vi "Charge and Discharge State Machine VI.vi"() -> ()   [LabVIEW 2017]
uses:
  Downloads/VVWRA HMM/Globals.vi
panel:
  out "Refresh Battery SOC (%)":u8
  out "Power Needed (kW)":i32
  out "Refresh Battery Power (kW)":i32
  out "Discharge Battery Power (kW)":i32
  out "Discharge State":T1(ring)
  out "SCE_Power (kW)":i32
  out "Charge State":T1(ring)
  out "Discharging Battery SOC (%)":u8
  out "Charging Battery SOC (%)":u8
  out "Charge Battery Power (kW)":i32
  in  "Stop Button":bool
  # "Contact information: \nMatthew Scudder\nmatthew.scudderr@gmail.com\n773-306-9466"
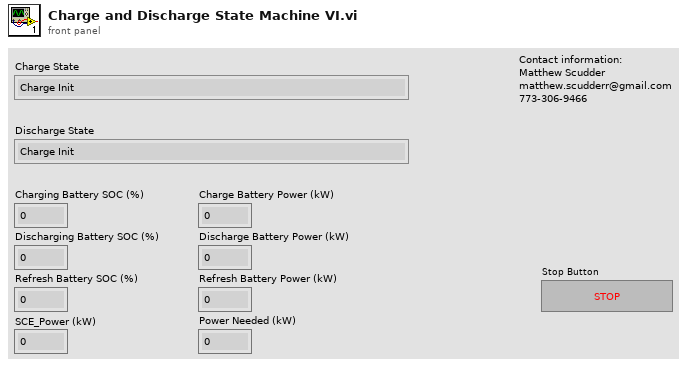
[diagram p1: front panel]
types:
  T1 = enum16{"Charge Init", "Start Charging Loop", "Check SOC < 75%", "Charge_Bat Power > -86 kW", "Charge_Bat Power = -86 kW", "Charge_Bat Power > -10 kW", "Discharge_Bat Power >= 40 kW && SCE_Power >= 110 kW", "Charge_Bat Power = Charge_Bat Power + 20kW", "Charge_Bat Power = 0 kW", "Wait for Discharge_Bat SOC", "Discharge Init", "Start Discharging Loop", "SCE_Power < 90 kW_1", "Discharge_Bat SOC < 25%_1", "Charge_Bat SOC >= 75%", "Battery Role Change", "SCE_Power < 95 kW_1", "Refresh_Bat Power = Refresh_Bat Power + 5 kW", "Refresh_Bat Power >= 100 kW", "Refresh_Bat SOC < 10%", "Refresh_Bat = Charge_Bat", "Power_Needed = 95 kW - SCE_Power", "Discharge_Bat Power - Power_Needed < -86 kW", "Alarm Discharge_Bat Can't Meet Demand", "Discharge_Bat Power = Discharge_Bat Power - Power_Needed", "SCE_Power < 90 kW_2", "SCE_Power < 95 kW_2", "Discharge_Bat Power = Discharge_Bat Power + 5 kW", "SCE_Power < 90 kW_3", "Discharge_Bat Power >= 40 kW", "Discharge_Bat SOC < 25%_2", "Shutdown"}
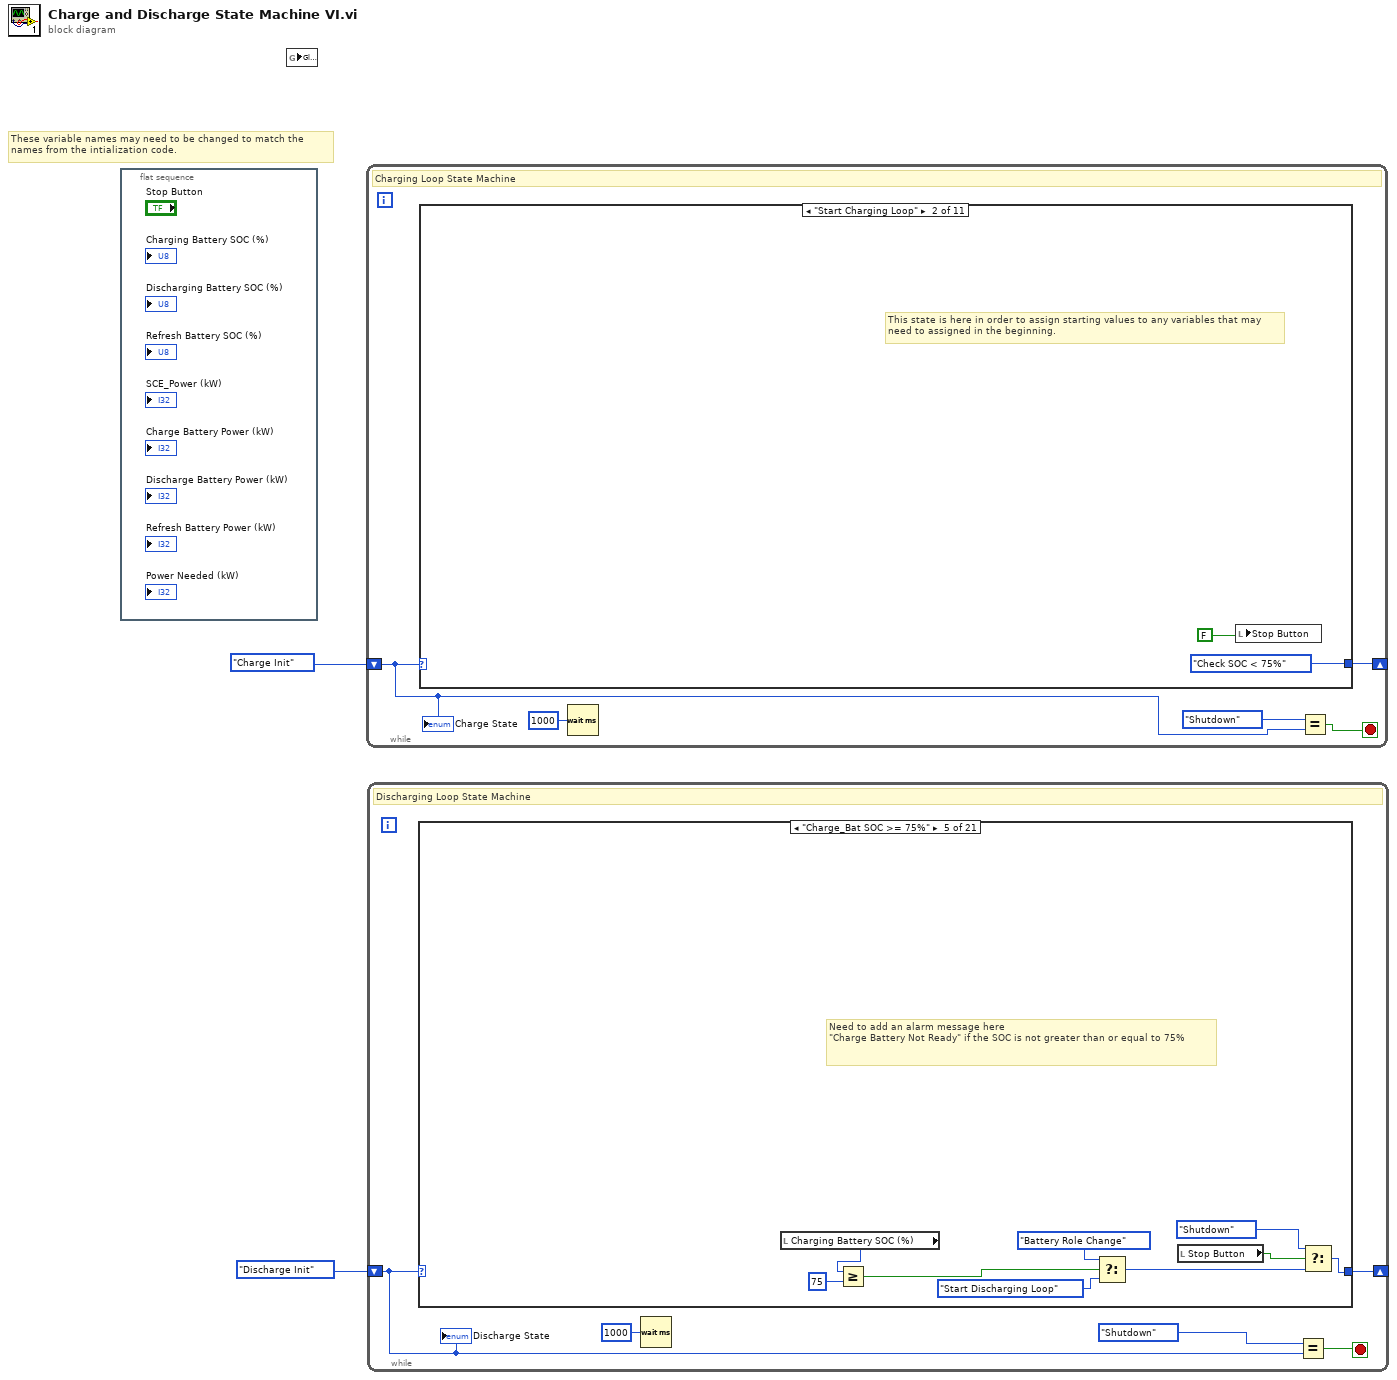
[diagram p0: block diagram]
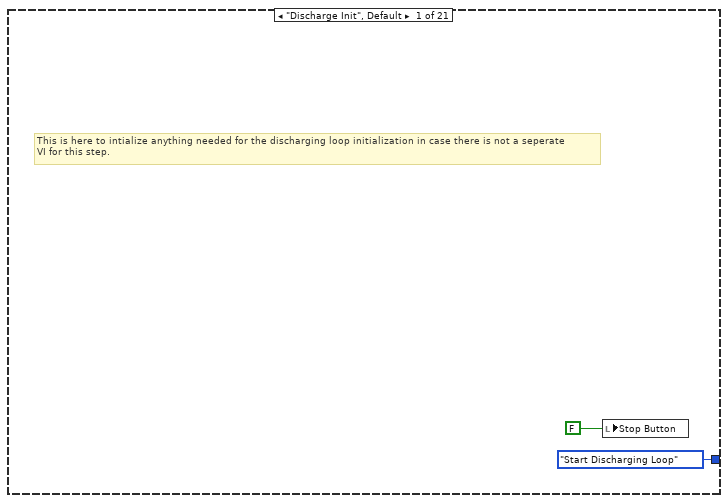
[diagram p2: hidden frame]
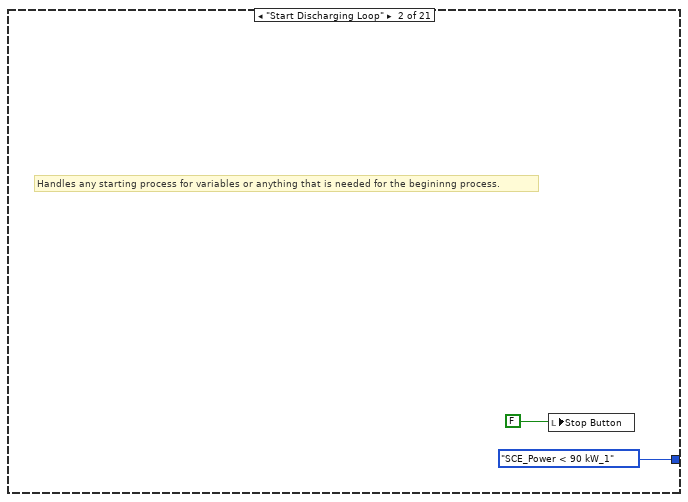
[diagram p3: hidden frame]
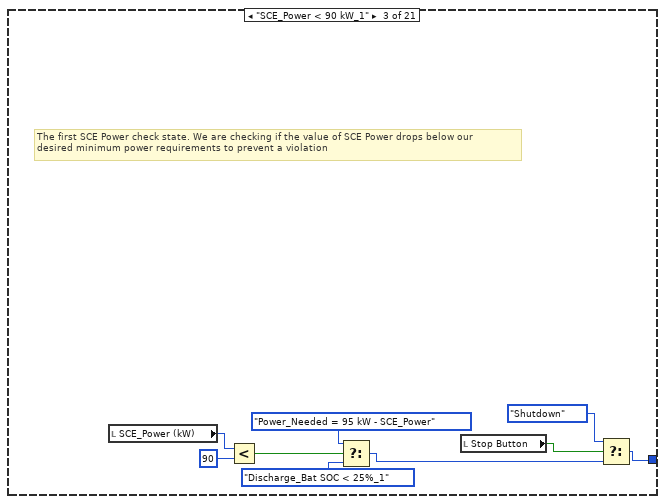
[diagram p4: hidden frame]
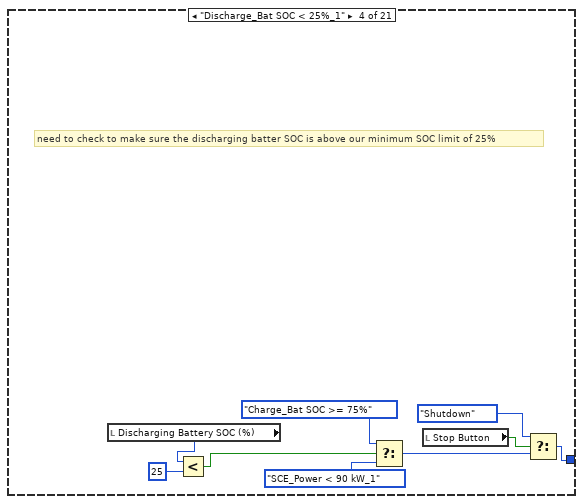
[diagram p5: hidden frame]
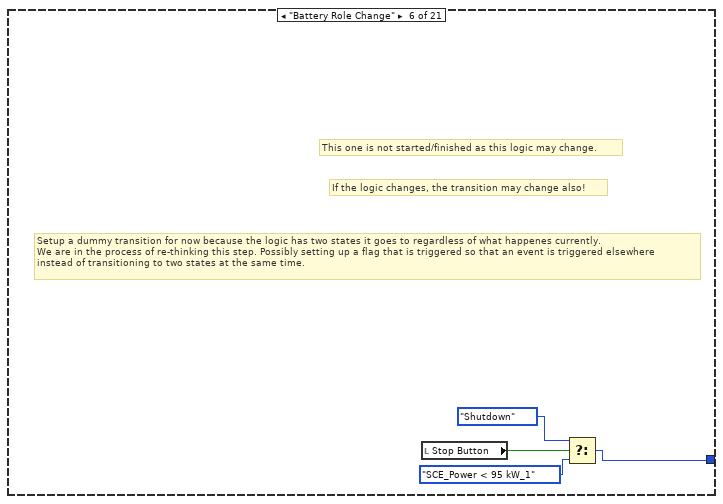
[diagram p6: hidden frame]
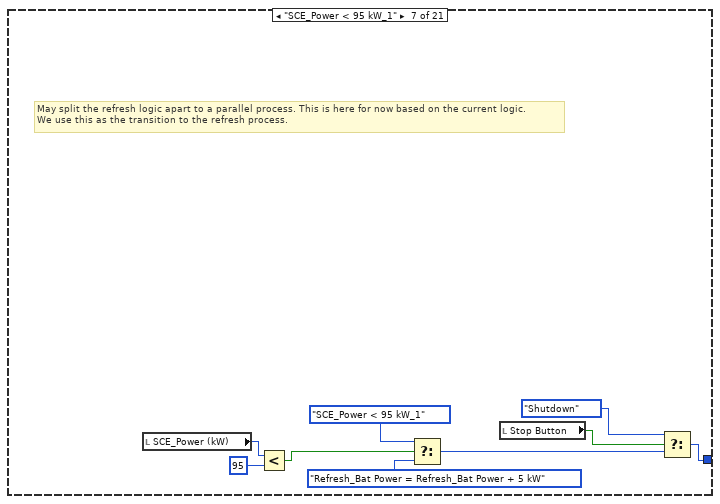
[diagram p7: hidden frame]
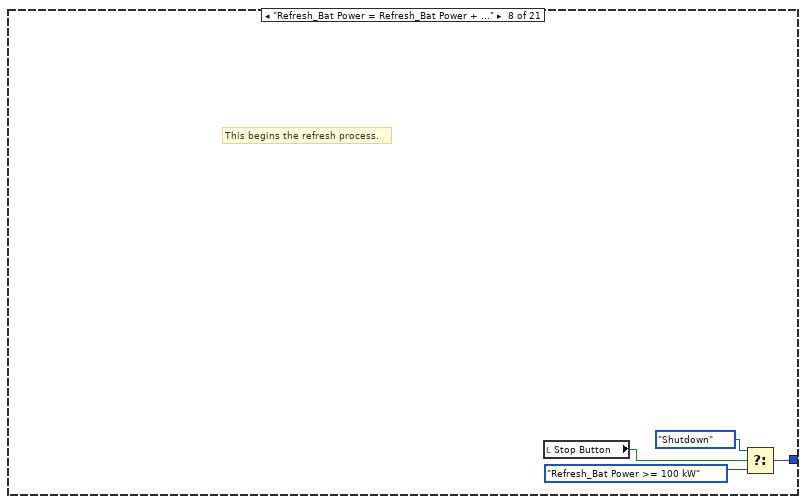
[diagram p8: hidden frame]
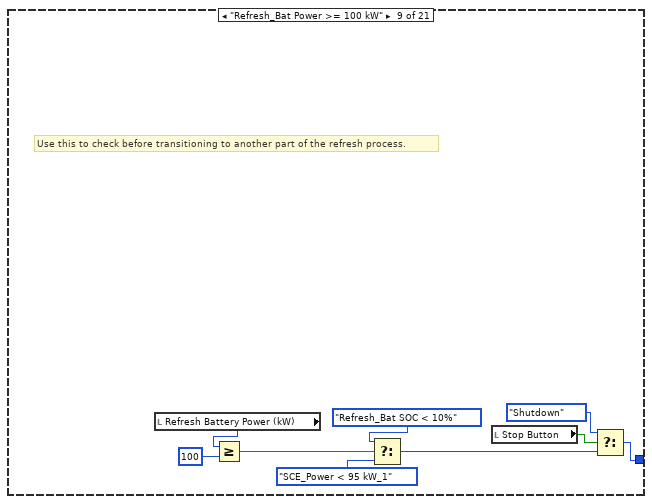
[diagram p9: hidden frame]
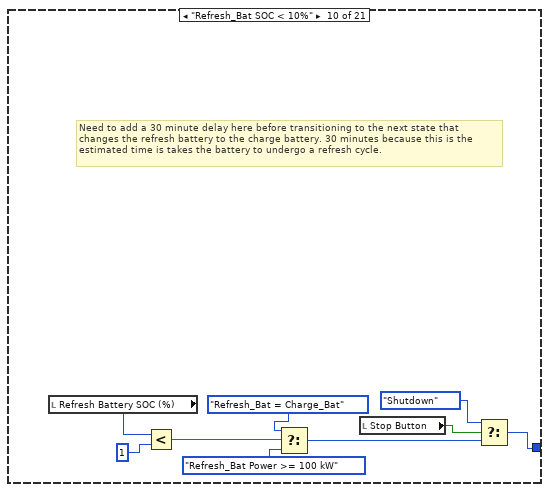
[diagram p10: hidden frame]
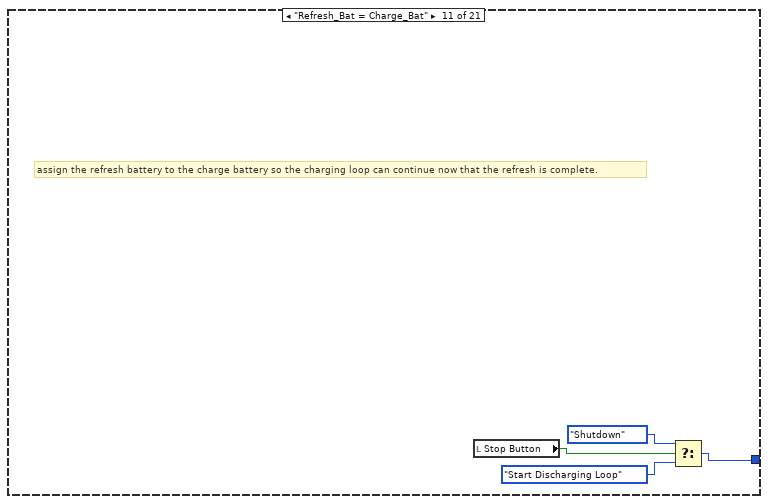
[diagram p11: hidden frame]
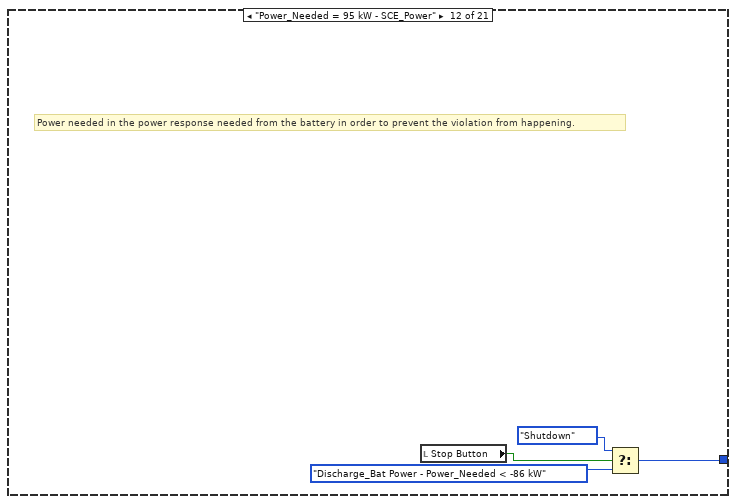
[diagram p12: hidden frame]
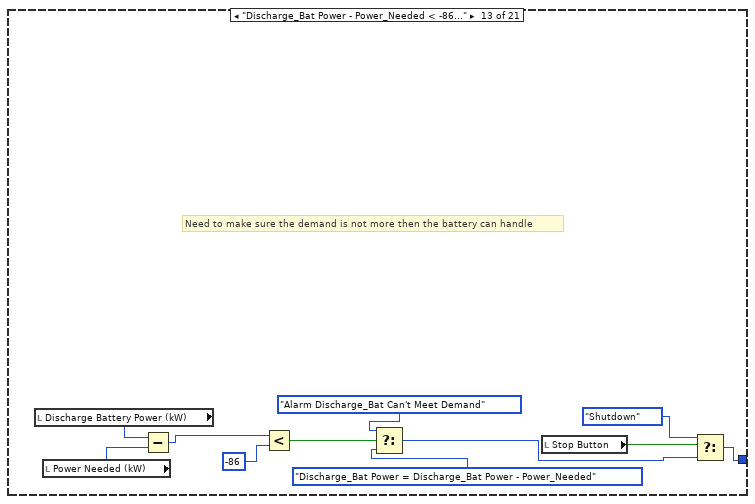
[diagram p13: hidden frame]
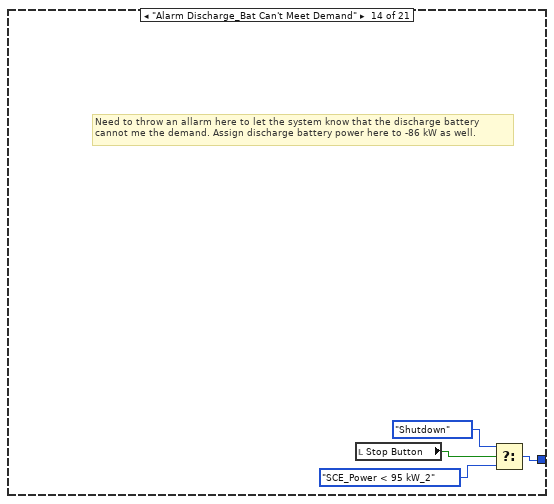
[diagram p14: hidden frame]
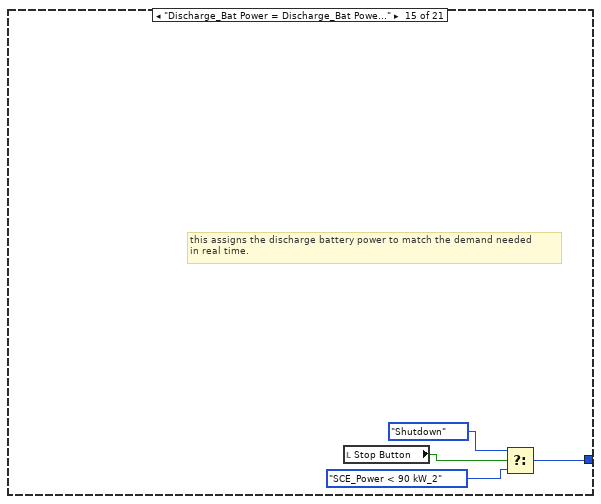
[diagram p15: hidden frame]
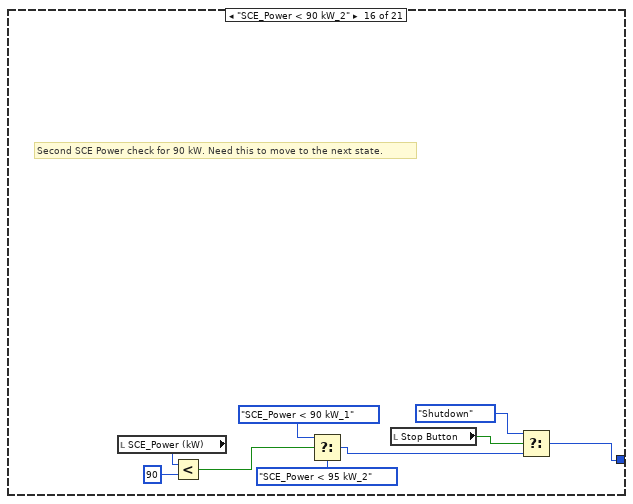
[diagram p16: hidden frame]
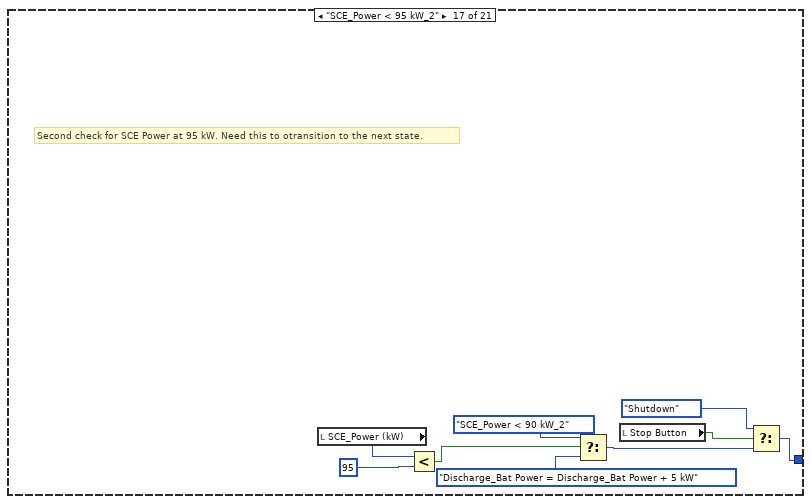
[diagram p17: hidden frame]
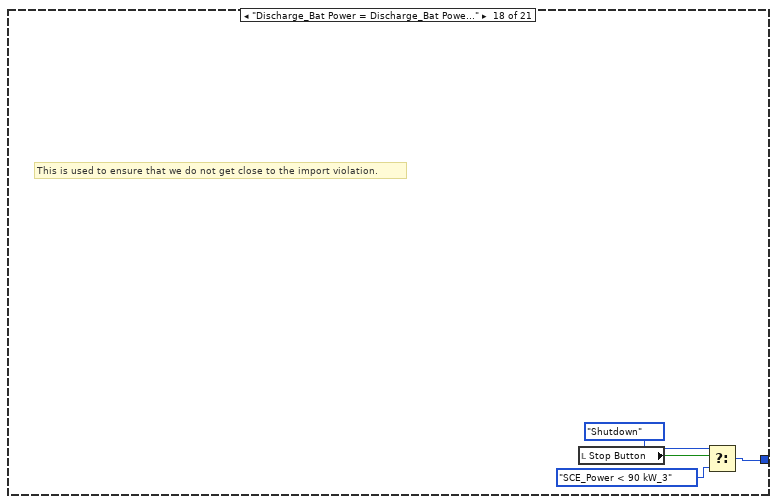
[diagram p18: hidden frame]
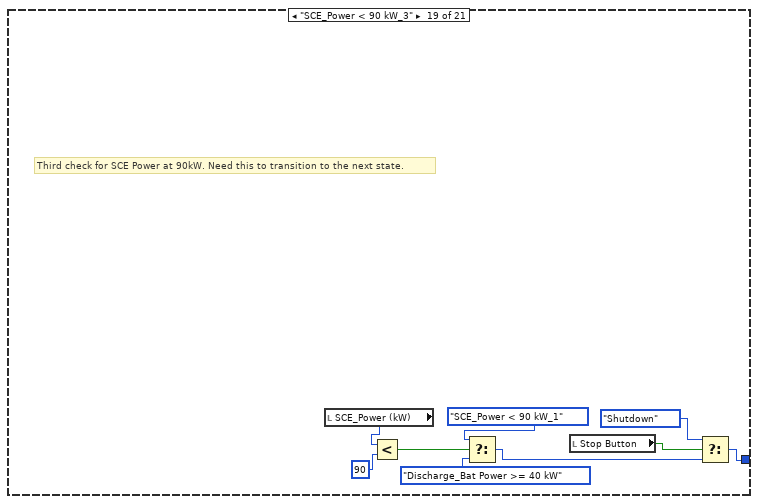
[diagram p19: hidden frame]
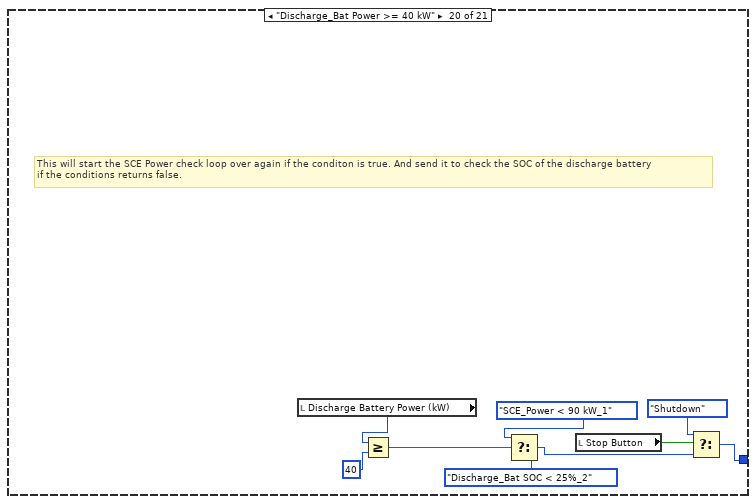
[diagram p20: hidden frame]
diagram:
  # "These variable names may need to be changed to match the \nnames from the intialization code."
  n1 = flat-sequence {
    frame #0 {
    }
  }
  n2 = global read "Globals.vi" item#-1() -> ()  [unwired: 1 in]
  n3 = while {
    shift-right: [w4] -> _
    shift-left: T1."Charge Init" ("States") -> [w5]
    stop <- w7 stop-if-true
    # "Charging Loop State Machine"
    n4 = case shown="\"Start Charging Loop\"" w5 {
      tunnel: [T1."Start Charging Loop" ("States") T1."Check SOC < 75%" ("States") w15 w22 w30 w34 w43 w59 w63 w72 T1."Shutdown" ("States")] -> w4
      frame "Charge Init", Default {
        # "Any Communication between the controller and the Inverters is done through a MODBUS Serial connection.\nThe inverter register values are in hex."
        # "Any communication between the controller and the BMS is done through MODBUS TCP/IP.\nThe BMS register values are in decimal."
        # "initialization code goes here. Either we use a subVI for the intitialization of the hardware or we \ninput the intialization code here."
        n5 = local write "Stop Button"(FALSE) -> ()
      }
      frame "Start Charging Loop" {
        # "This state is here in order to assign starting values to any variables that may\nneed to assigned in the beginning."
        n6 = local write "Stop Button"(FALSE) -> ()
      }
      frame "Check SOC < 75%" {
        # "We need to read in values of the battery that is currently assigned to charge. This is done using MODBUS TCP/IP\nbetween our controller and the BMS of the charging battery. The maximum allowed SOC is 75%"
        n7 = local read "Charging Battery SOC (%)"() -> (w20:u8)
        n8 = Less?(x=w20, y=u8 75) -> (x < y?=w18:bool)
        n9 = Select(t=T1."Charge_Bat Power > -86 kW" ("States"), s=w18, f=T1."Charge_Bat Power > -10 kW" ("States")) -> (s? t:f=w13:T1)
        n10 = local read "Stop Button"() -> (w12:bool)
        n11 = Select(t=T1."Shutdown" ("States"), s=w12, f=w13) -> (s? t:f=w15:T1)
      }
      frame "Charge_Bat Power > -86 kW" {
        # "We need the charging battery output power to be set to -86 kW here because of the requirements of the \ntypes of batteries that we are working with.\nThis is used to keep the battery within the SOC limit range of 25%-75%"
        n12 = local read "Charge Battery Power (kW)"() -> (w25:i32)
        n13 = Greater?(x=w25, y=-86) -> (0:w24:bool)
        n14 = Select(t=T1."Charge_Bat Power = -86 kW" ("States"), s=w24, f=T1."Check SOC < 75%" ("States")) -> (s? t:f=w26:T1)
        n15 = local read "Stop Button"() -> (w21:bool)
        n16 = Select(t=T1."Shutdown" ("States"), s=w21, f=w26) -> (s? t:f=w22:T1)
      }
      frame "Charge_Bat Power = -86 kW" {
        # "We need to discharge the battery to 75% SOC if it is over 75% SOC"
        n17 = local read "Stop Button"() -> (w33:bool)
        n18 = Select(t=T1."Shutdown" ("States"), s=w33, f=T1."Check SOC < 75%" ("States")) -> (s? t:f=w30:T1)
      }
      frame "Charge_Bat Power > -10 kW" {
        # "We use this check to either send the battery into a dwell state that waits for the discharge battery \nor another check that compares both the SCE power and discharge battery output"
        n19 = local read "Charge Battery Power (kW)"() -> (w42:i32)
        n20 = Greater?(x=w42, y=-10) -> (0:w40:bool)
        n21 = Select(t=T1."Charge_Bat Power = 0 kW" ("States"), s=w40, f=T1."Discharge_Bat Power >= 40 kW && SCE_Power >= 110 kW" ("States")) -> (s? t:f=w37:T1)
        n22 = local read "Stop Button"() -> (w36:bool)
        n23 = Select(t=T1."Shutdown" ("States"), s=w36, f=w37) -> (s? t:f=w34:T1)
      }
      frame "Discharge_Bat Power >= 40 kW && SCE_Power >= 110 kW" {
        # "We need to check if both the SCE Power and Discharge Battery Power conditions are met in order\nto move to the next state. We will continue to stay in this state until the conditions are met"
        n24 = local read "Discharge Battery Power (kW)"() -> (w55:i32)
        n25 = local read "SCE_Power (kW)"() -> (w52:i32)
        n26 = Greater Or Equal?(x=w55, y=40) -> (x >= y?=w53:bool)
        n27 = Greater Or Equal?(x=w52, y=110) -> (x >= y?=w50:bool)
        n28 = And(x=w53, y=w50) -> (x .and. y?=w49:bool)
        n29 = Select(t=T1."Charge_Bat Power = Charge_Bat Power + 20kW" ("States"), s=w49, f=T1."Discharge_Bat Power >= 40 kW && SCE_Power >= 110 kW" ("States")) -> (s? t:f=w46:T1)
        n30 = local read "Stop Button"() -> (w45:bool)
        n31 = Select(t=T1."Shutdown" ("States"), s=w45, f=w46) -> (s? t:f=w43:T1)
      }
      frame "Charge_Bat Power = Charge_Bat Power + 20kW" {
        # "Need add a 30 delay here before moving onto the next state"
        n32 = local read "Stop Button"() -> (w56:bool)
        n33 = Select(t=T1."Shutdown" ("States"), s=w56, f=T1."Charge_Bat Power > -10 kW" ("States")) -> (s? t:f=w59:T1)
      }
      frame "Charge_Bat Power = 0 kW" {
        # "We need to set the charging battery to zerro output and input in order to wait for the discharging battery SOC"
        n34 = local read "Stop Button"() -> (w60:bool)
        n35 = Select(t=T1."Shutdown" ("States"), s=w60, f=T1."Wait for Discharge_Bat SOC" ("States")) -> (s? t:f=w63:T1)
      }
      frame "Wait for Discharge_Bat SOC" {
        # "The charging loop can begin again once the discharging battery reaches 0% SOC making the discharge battery \nswitch to the refresh battery and the charging battery switch to a discharging battery."
        n36 = local read "Discharging Battery SOC (%)"() -> (w66:u8)
        n37 = Equal?(x=w66, y=u8 0) -> (x = y?=w64:bool)
        n38 = Select(t=T1."Start Charging Loop" ("States"), s=w64, f=T1."Wait for Discharge_Bat SOC" ("States")) -> (s? t:f=w69:T1)
        n39 = local read "Stop Button"() -> (w70:bool)
        n40 = Select(t=T1."Shutdown" ("States"), s=w70, f=w69) -> (s? t:f=w72:T1)
      }
      frame "Shutdown" {
        # "Have this state in cause the system needs to be shut down in a certain order as to save any variable data that would be \nnecessary for the initialzation of the program once booted up again."
      }
    }
    n41 = Wait (ms)(milliseconds to wait=u32 1000) -> ()  [unwired: 1 out]
    n42 = Equal?(x=T1."Shutdown" ("States"), y=w5) -> (x = y?=w7:bool)
    "Charge State" <- w5
  }
  n43 = while {
    shift-right: [w75] -> _
    shift-left: T1."Discharge Init" ("States") -> [w77]
    stop <- w78 stop-if-true
    # "Discharging Loop State Machine"
    n44 = case shown="\"Charge_Bat SOC >= 75%\"" w77 {
      tunnel: [T1."Start Discharging Loop" ("States") T1."SCE_Power < 90 kW_1" ("States") w83 w92 w102 w113 w114 w123 w127 w136 w145 w152 w153 w167 w171 w172 w181 w190 w194 w203 w212] -> w75
      frame "Discharge Init", Default {
        # "This is here to intialize anything needed for the discharging loop initialization in case there is not a seperate\nVI for this step."
        n45 = local write "Stop Button"(FALSE) -> ()
      }
      frame "Start Discharging Loop" {
        # "Handles any starting process for variables or anything that is needed for the begininng process."
        n46 = local write "Stop Button"(FALSE) -> ()
      }
      frame "SCE_Power < 90 kW_1" {
        # "The first SCE Power check state. We are checking if the value of SCE Power drops below our \ndesired minimum power requirements to prevent a violation"
        n47 = local read "SCE_Power (kW)"() -> (w91:i32)
        n48 = Less?(x=w91, y=90) -> (x < y?=w89:bool)
        n49 = Select(t=T1."Power_Needed = 95 kW - SCE_Power" ("States"), s=w89, f=T1."Discharge_Bat SOC < 25%_1" ("States")) -> (s? t:f=w86:T1)
        n50 = local read "Stop Button"() -> (w85:bool)
        n51 = Select(t=T1."Shutdown" ("States"), s=w85, f=w86) -> (s? t:f=w83:T1)
      }
      frame "Discharge_Bat SOC < 25%_1" {
        # "need to check to make sure the discharging batter SOC is above our minimum SOC limit of 25%"
        n52 = local read "Discharging Battery SOC (%)"() -> (w100:u8)
        n53 = Less?(x=w100, y=u8 25) -> (x < y?=w98:bool)
        n54 = Select(t=T1."Charge_Bat SOC >= 75%" ("States"), s=w98, f=T1."SCE_Power < 90 kW_1" ("States")) -> (s? t:f=w95:T1)
        n55 = local read "Stop Button"() -> (w94:bool)
        n56 = Select(t=T1."Shutdown" ("States"), s=w94, f=w95) -> (s? t:f=w92:T1)
      }
      frame "Charge_Bat SOC >= 75%" {
        # "Need to add an alarm message here\n\"Charge Battery Not Ready\" if the SOC is not greater than or equal to 75%"
        n57 = local read "Charging Battery SOC (%)"() -> (w109:u8)
        n58 = Greater Or Equal?(x=w109, y=u8 75) -> (x >= y?=w107:bool)
        n59 = Select(t=T1."Battery Role Change" ("States"), s=w107, f=T1."Start Discharging Loop" ("States")) -> (s? t:f=w105:T1)
        n60 = local read "Stop Button"() -> (w103:bool)
        n61 = Select(t=T1."Shutdown" ("States"), s=w103, f=w105) -> (s? t:f=w102:T1)
      }
      frame "Battery Role Change" {
        # "Setup a dummy transition for now because the logic has two states it goes to regardless of what happenes currently.\nWe are in the process of re-thinking this step. Possibly setting up a flag that is triggered so that an event is triggered elsewhere\ninstead of transitioning to two states at the same time."
        # "If the logic changes, the transition may change also!"
        # "This one is not started/finished as this logic may change."
        n62 = local read "Stop Button"() -> (w111:bool)
        n63 = Select(t=T1."Shutdown" ("States"), s=w111, f=T1."SCE_Power < 95 kW_1" ("States")) -> (s? t:f=w113:T1)
      }
      frame "SCE_Power < 95 kW_1" {
        # "May split the refresh logic apart to a parallel process. This is here for now based on the current logic.\nWe use this as the transition to the refresh process."
        n64 = local read "SCE_Power (kW)"() -> (w121:i32)
        n65 = Less?(x=w121, y=95) -> (x < y?=w120:bool)
        n66 = Select(t=T1."SCE_Power < 95 kW_1" ("States"), s=w120, f=T1."Refresh_Bat Power = Refresh_Bat Power + 5 kW" ("States")) -> (s? t:f=w117:T1)
        n67 = local read "Stop Button"() -> (w116:bool)
        n68 = Select(t=T1."Shutdown" ("States"), s=w116, f=w117) -> (s? t:f=w114:T1)
      }
      frame "Refresh_Bat Power = Refresh_Bat Power + 5 kW" {
        # "This begins the refresh process."
        n69 = local read "Stop Button"() -> (w125:bool)
        n70 = Select(t=T1."Shutdown" ("States"), s=w125, f=T1."Refresh_Bat Power >= 100 kW" ("States")) -> (s? t:f=w123:T1)
      }
      frame "Refresh_Bat Power >= 100 kW" {
        # "Use this to check before transitioning to another part of the refresh process."
        n71 = local read "Refresh Battery Power (kW)"() -> (w135:i32)
        n72 = Greater Or Equal?(x=w135, y=100) -> (x >= y?=w133:bool)
        n73 = Select(t=T1."Refresh_Bat SOC < 10%" ("States"), s=w133, f=T1."SCE_Power < 95 kW_1" ("States")) -> (s? t:f=w130:T1)
        n74 = local read "Stop Button"() -> (w129:bool)
        n75 = Select(t=T1."Shutdown" ("States"), s=w129, f=w130) -> (s? t:f=w127:T1)
      }
      frame "Refresh_Bat SOC < 10%" {
        # "Need to add a 30 minute delay here before transitioning to the next state that \nchanges the refresh battery to the charge battery. 30 minutes because this is the \nestimated time is takes the battery to undergo a refresh cycle."
        n76 = local read "Refresh Battery SOC (%)"() -> (w144:u8)
        n77 = Less?(x=w144, y=u8 1) -> (x < y?=w142:bool)
        n78 = Select(t=T1."Refresh_Bat = Charge_Bat" ("States"), s=w142, f=T1."Refresh_Bat Power >= 100 kW" ("States")) -> (s? t:f=w139:T1)
        n79 = local read "Stop Button"() -> (w138:bool)
        n80 = Select(t=T1."Shutdown" ("States"), s=w138, f=w139) -> (s? t:f=w136:T1)
      }
      frame "Refresh_Bat = Charge_Bat" {
        # "assign the refresh battery to the charge battery so the charging loop can continue now that the refresh is complete."
        n81 = local read "Stop Button"() -> (w147:bool)
        n82 = Select(t=T1."Shutdown" ("States"), s=w147, f=T1."Start Discharging Loop" ("States")) -> (s? t:f=w145:T1)
      }
      frame "Power_Needed = 95 kW - SCE_Power" {
        # "Power needed in the power response needed from the battery in order to prevent the violation from happening."
        n83 = local read "Stop Button"() -> (w150:bool)
        n84 = Select(t=T1."Shutdown" ("States"), s=w150, f=T1."Discharge_Bat Power - Power_Needed < -86 kW" ("States")) -> (s? t:f=w152:T1)
      }
      frame "Discharge_Bat Power - Power_Needed < -86 kW" {
        # "Need to make sure the demand is not more then the battery can handle"
        n85 = local read "Discharge Battery Power (kW)"() -> (w163:i32)
        n86 = local read "Power Needed (kW)"() -> (w162:i32)
        n87 = Subtract(x=w163, y=w162) -> (x-y=w161:i32)
        n88 = Less?(x=w161, y=-86) -> (x < y?=w159:bool)
        n89 = Select(t=T1."Alarm Discharge_Bat Can't Meet Demand" ("States"), s=w159, f=T1."Discharge_Bat Power = Discharge_Bat Power - Power_Needed" ("States")) -> (s? t:f=w154:T1)
        n90 = local read "Stop Button"() -> (w155:bool)
        n91 = Select(t=T1."Shutdown" ("States"), s=w155, f=w154) -> (s? t:f=w153:T1)
      }
      frame "Alarm Discharge_Bat Can't Meet Demand" {
        # "Need to throw an allarm here to let the system know that the discharge battery \ncannot me the demand. Assign discharge battery power here to -86 kW as well."
        n92 = local read "Stop Button"() -> (w166:bool)
        n93 = Select(t=T1."Shutdown" ("States"), s=w166, f=T1."SCE_Power < 95 kW_2" ("States")) -> (s? t:f=w167:T1)
      }
      frame "Discharge_Bat Power = Discharge_Bat Power - Power_Needed" {
        # "this assigns the discharge battery power to match the demand needed\nin real time."
        n94 = local read "Stop Button"() -> (w170:bool)
        n95 = Select(t=T1."Shutdown" ("States"), s=w170, f=T1."SCE_Power < 90 kW_2" ("States")) -> (s? t:f=w171:T1)
      }
      frame "SCE_Power < 90 kW_2" {
        # "Second SCE Power check for 90 kW. Need this to move to the next state."
        n96 = local read "SCE_Power (kW)"() -> (w180:i32)
        n97 = Less?(x=w180, y=90) -> (x < y?=w178:bool)
        n98 = Select(t=T1."SCE_Power < 90 kW_1" ("States"), s=w178, f=T1."SCE_Power < 95 kW_2" ("States")) -> (s? t:f=w175:T1)
        n99 = local read "Stop Button"() -> (w174:bool)
        n100 = Select(t=T1."Shutdown" ("States"), s=w174, f=w175) -> (s? t:f=w172:T1)
      }
      frame "SCE_Power < 95 kW_2" {
        # "Second check for SCE Power at 95 kW. Need this to otransition to the next state."
        n101 = local read "SCE_Power (kW)"() -> (w189:i32)
        n102 = Less?(x=w189, y=95) -> (x < y?=w187:bool)
        n103 = Select(t=T1."SCE_Power < 90 kW_2" ("States"), s=w187, f=T1."Discharge_Bat Power = Discharge_Bat Power + 5 kW" ("States")) -> (s? t:f=w184:T1)
        n104 = local read "Stop Button"() -> (w183:bool)
        n105 = Select(t=T1."Shutdown" ("States"), s=w183, f=w184) -> (s? t:f=w181:T1)
      }
      frame "Discharge_Bat Power = Discharge_Bat Power + 5 kW" {
        # "This is used to ensure that we do not get close to the import violation."
        n106 = local read "Stop Button"() -> (w193:bool)
        n107 = Select(t=T1."Shutdown" ("States"), s=w193, f=T1."SCE_Power < 90 kW_3" ("States")) -> (s? t:f=w190:T1)
      }
      frame "SCE_Power < 90 kW_3" {
        # "Third check for SCE Power at 90kW. Need this to transition to the next state."
        n108 = local read "SCE_Power (kW)"() -> (w202:i32)
        n109 = Less?(x=w202, y=90) -> (x < y?=w200:bool)
        n110 = Select(t=T1."SCE_Power < 90 kW_1" ("States"), s=w200, f=T1."Discharge_Bat Power >= 40 kW" ("States")) -> (s? t:f=w197:T1)
        n111 = local read "Stop Button"() -> (w196:bool)
        n112 = Select(t=T1."Shutdown" ("States"), s=w196, f=w197) -> (s? t:f=w194:T1)
      }
      frame "Discharge_Bat Power >= 40 kW" {
        # "This will start the SCE Power check loop over again if the conditon is true. And send it to check the SOC of the discharge battery \nif the conditions returns false."
        n113 = local read "Discharge Battery Power (kW)"() -> (w211:i32)
        n114 = Greater Or Equal?(x=w211, y=40) -> (x >= y?=w209:bool)
        n115 = Select(t=T1."SCE_Power < 90 kW_1" ("States"), s=w209, f=T1."Discharge_Bat SOC < 25%_2" ("States")) -> (s? t:f=w206:T1)
        n116 = local read "Stop Button"() -> (w205:bool)
        n117 = Select(t=T1."Shutdown" ("States"), s=w205, f=w206) -> (s? t:f=w203:T1)
      }
      frame "Discharge_Bat SOC < 25%_2" {
        # "If the condition is true we need to check the charging battery  SOC again to see if a role change is needed.\nIf not, we go back to checking the SCE Power again."
        n118 = local read "Discharging Battery SOC (%)"() -> (w220:u8)
        n119 = Less?(x=w220, y=u8 25) -> (x < y?=w218:bool)
        n120 = Select(t=T1."Charge_Bat SOC >= 75%" ("States"), s=w218, f=T1."SCE_Power < 95 kW_2" ("States")) -> (s? t:f=w215:T1)
        n121 = local read "Stop Button"() -> (w214:bool)
        n122 = Select(t=T1."Shutdown" ("States"), s=w214, f=w215) -> (s? t:f=w212:T1)
      }
    }
    n123 = Wait (ms)(milliseconds to wait=u32 1000) -> ()  [unwired: 1 out]
    n124 = Equal?(x=T1."Shutdown" ("States"), y=w77) -> (x = y?=w78:bool)
    "Discharge State" <- w77
  }
